vi "Read & Update TimerCounter Values.vi"(0 "Handle In":i32, 1 "Reset Counter0":bool, 2 "Reset Counter1":bool, 5 "# Timers to Read":i32, 7 "UpdateReset Timers":bool[](array[boolean])=[FALSE, FALSE, FALSE, FALSE, FALSE, FALSE], 9 "TimerValues":dbl[](array[numeric])=[0.0, 0.0, 0.0, 0.0, 0.0, 0.0] format="%.2f", 11 "error in":errorcluster, 12 "Read Counter0":bool, 13 "Read Counter1":bool) -> (4 "Handle Out":i32, 6 "Timer Value Reads":dbl[](array[numeric]) format="%.2f", 8 "Counter Value Reads":dbl[](array[numeric]) format="%.2f", 15 "error out":errorcluster)   [LabVIEW 2021]
panel:
  # "Determines which, if any, timers are updated/reset."
  # "Counter0\n\nCounter1"
  # "Always returns 2 elements,\neven if only 1 counter is\nread."
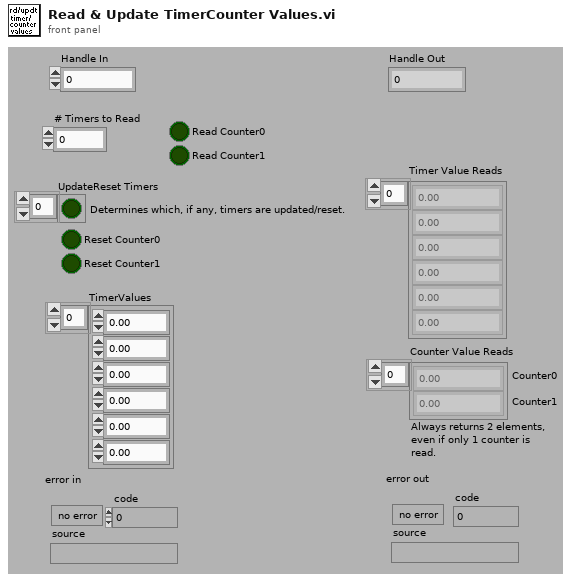
[diagram p1: front panel]
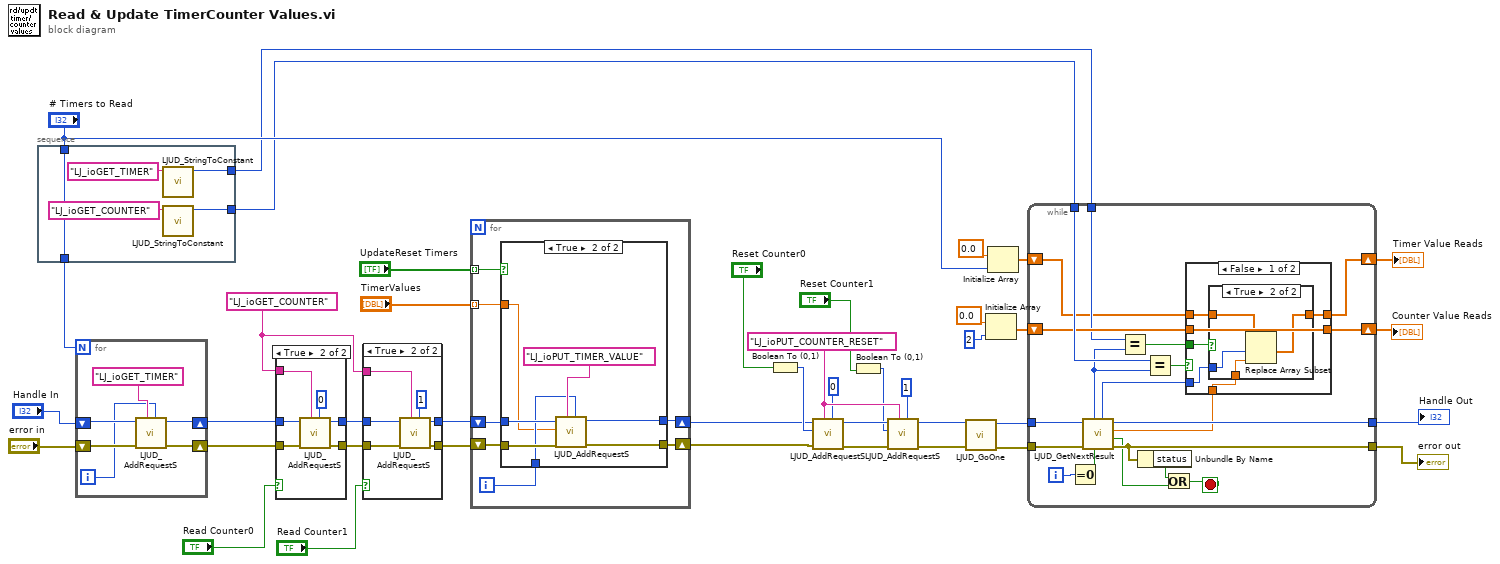
[diagram p0: block diagram]
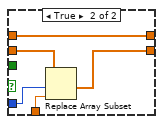
[diagram p3: hidden frame]
diagram:
  w37 = "LJ_ioPUT_COUNTER_RESET" ("IOType")
  w3 = "LJ_ioGET_COUNTER" ("IOType")
  n1 = stacked-sequence {
    tunnel: "# Timers to Read" -> [w44]
    tunnel: [w44] -> w24
    tunnel: [w43] -> w10
    tunnel: [w42] -> w11
    frame #0 {
      n2 = call "LJUD_StringToConstant.vi"("String"="LJ_ioGET_TIMER" ("IOType")) -> ("Constant Number"=w43:i32)  [unwired: 9 in, 1 out]
      n3 = call "LJUD_StringToConstant.vi"("String"="LJ_ioGET_COUNTER" ("IOType")) -> ("Constant Number"=w42:i32)  [unwired: 9 in, 1 out]
    }
  }
  n4 = for {
    N: w24 -> [_]
    shift-right: [w47] -> w27
    shift-left: "error in" -> [w51]
    shift-right: [w48] -> w28
    shift-left: "Handle In" -> [w50]
    i -> [w49]
    n5 = call "LJUD_AddRequestS.vi"("Channel"=w49, "IOType"="LJ_ioGET_TIMER", "error in"=w51, "Handle In"=w50) -> ("error out"=w47:errorcluster, "Handle Out"=w48:i32)  [unwired: 6 in]
  }
  n6 = case shown="True" "Read Counter0" {
    tunnel: w3 -> [_ w55]
    tunnel: [w53 w59] -> w41
    tunnel: [w54 w58] -> w40
    tunnel: w28 -> [w54 w57]
    tunnel: w27 -> [w53 w56]
    frame False {
    }
    frame True {
      n7 = call "LJUD_AddRequestS.vi"("Channel"=0, "IOType"=w55, "error in"=w56, "Handle In"=w57) -> ("error out"=w59:errorcluster, "Handle Out"=w58:i32)  [unwired: 6 in]
    }
  }
  n8 = case shown="True" "Read Counter1" {
    tunnel: w3 -> [_ w67]
    tunnel: w41 -> [w61 w66]
    tunnel: w40 -> [w62 w65]
    tunnel: [w61 w64] -> w7
    tunnel: [w62 w63] -> w6
    frame False {
    }
    frame True {
      n9 = call "LJUD_AddRequestS.vi"("Channel"=1, "IOType"=w67, "error in"=w66, "Handle In"=w65) -> ("error out"=w64:errorcluster, "Handle Out"=w63:i32)  [unwired: 6 in]
    }
  }
  n10 = for {
    tunnel: "UpdateReset Timers" -> [w75] mode=indexing
    tunnel: "TimerValues" -> [w73] mode=indexing
    shift-right: [w69] -> w5
    shift-left: w6 -> [w70]
    shift-right: [w71] -> w4
    shift-left: w7 -> [w72]
    i -> [w74]
    n11 = case shown="True" w75 {
      tunnel: w70 -> [w77 w83]
      tunnel: w72 -> [w76 w82]
      tunnel: w74 -> [_ w81]
      tunnel: w73 -> [_ w80]
      tunnel: [w76 w79] -> w71
      tunnel: [w77 w78] -> w69
      frame False {
      }
      frame True {
        n12 = call "LJUD_AddRequestS.vi"("Channel"=w81, "IOType"="LJ_ioPUT_TIMER_VALUE", "error in"=w82, "Value"=w80, "Handle In"=w83) -> ("error out"=w79:errorcluster, "Handle Out"=w78:i32)  [unwired: 5 in]
      }
    }
  }
  n13 = Boolean To (0,1)(Boolean="Reset Counter0") -> (0, 1=w31:i16)
  n14 = call "LJUD_AddRequestS.vi"("Channel"=0, "IOType"=w37, "error in"=w4, "Value"=w31, "Handle In"=w5) -> ("error out"=w39:errorcluster, "Handle Out"=w38:i32)  [unwired: 5 in]
  n15 = Boolean To (0,1)(Boolean="Reset Counter1") -> (0, 1=w33:i16)
  n16 = call "LJUD_AddRequestS.vi"("Channel"=1, "IOType"=w37, "error in"=w39, "Value"=w33, "Handle In"=w38) -> ("error out"=w26:errorcluster, "Handle Out"=w25:i32)  [unwired: 5 in]
  n17 = call "LJUD_GoOne.vi"("error in"=w26, "Handle In"=w25) -> ("error out"=w14:errorcluster, "Handle Out"=w15:i32)  [unwired: 8 in]
  n18 = Initialize Array(0.0 ("Channel"), 2 ("Channel")) -> (w19:dbl[])
  n19 = Initialize Array(0.0 ("Channel"), "# Timers to Read") -> (w17:dbl[])
  n20 = while {
    tunnel: w10 -> [w88]
    shift-left: w17 -> [w86]
    shift-right: [w85] -> w12
    shift-left: w19 -> [w92]
    shift-right: [w91] -> w13
    tunnel: w11 -> [w94]
    tunnel: [w98] -> w23
    tunnel: [w100] -> w22
    tunnel: w15 -> [w101]
    tunnel: w14 -> [w102]
    i -> [w97]
    stop <- w104 stop-if-true
    n21 = Equal To 0?(x=w97) -> (x = 0?=w103:bool)
    n22 = call "LJUD_GetNextResult.vi"("GetFirst"=w103, "error in"=w102, "Handle In"=w101) -> ("error out"=w100:errorcluster, "LJE_NO_MORE_DATA_AVAILABLE"=w96:bool, "Value"=w95:dbl, "Handle Out"=w98:i32, "Channel"=w90:i32, "IOType"=w89:i32)  [unwired: 3 in]
    n23 = Equal?(x=w88, y=w89) -> (x = y?=w87:bool)
    n24 = Unbundle By Name(w100) -> ("status"=w99:bool)
    n25 = Equal?(x=w94, y=w89) -> (x = y?=w93:bool)
    n26 = Or(x=w99, y=w96) -> (x .or. y?=w104:bool)
    n27 = case shown="False" w93 {
      tunnel: w95 -> [w108 w119]
      tunnel: w90 -> [w107 w120]
      tunnel: w92 -> [w105 w118]
      tunnel: [w105 w117] -> w91
      tunnel: w87 -> [w110 _]
      tunnel: w86 -> [w109 w116]
      tunnel: [w106 w116] -> w85
      frame False {
        n28 = case shown="True" w110 {
          tunnel: w108 -> [_ w114]
          tunnel: w107 -> [_ w115]
          tunnel: w109 -> [w111 w113]
          tunnel: [w111 w112] -> w106
          frame False {
          }
          frame True {
            n29 = Replace Array Subset(array=w113, new element=w114, index=w115) -> (w112:dbl[])
          }
        }
      }
      frame True {
        n30 = Replace Array Subset(array=w118, new element=w119, index=w120) -> (w117:dbl[])
      }
    }
  }
  "error out" <- w22
  "Handle Out" <- w23
  "Timer Value Reads" <- w12
  "Counter Value Reads" <- w13
